vi "DriveForDistance.vi"() -> ()   [LabVIEW 2018]
uses:
  Framework/Robot Global Data.vi
panel:
  in  "NoWait":bool
  in  "Speed":dbl
  in  "Distance":dbl
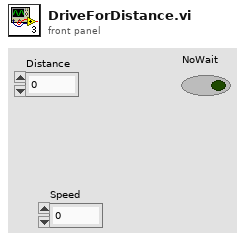
[diagram p1: front panel]
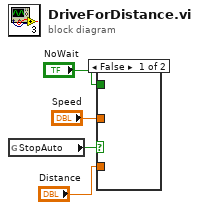
[diagram p0: block diagram]
diagram:
  n1 = global read "Robot Global Data.vi" "StopAuto"() -> (w1:bool)
  n2 = case shown="False" w1 {
    tunnel: "Distance" -> [_ _]
    tunnel: "Speed" -> [_ _]
    tunnel: "NoWait" -> [_ _]
    frame False {
    }
    frame True {
    }
  }
